vi "view variant in tree helper.vi"(4 "is array element?":bool, 5 "is attribute?":bool, 6 "index string":string, 7 "name":string, 8 "error in (no error)":errorcluster, 9 "Item Indent":i32, 10 "Variant":variant, 11 "Items":T1(array[cluster])) -> (0 "error out":errorcluster, 3 "Items out":T1(array[cluster]))   [LabVIEW 2016]
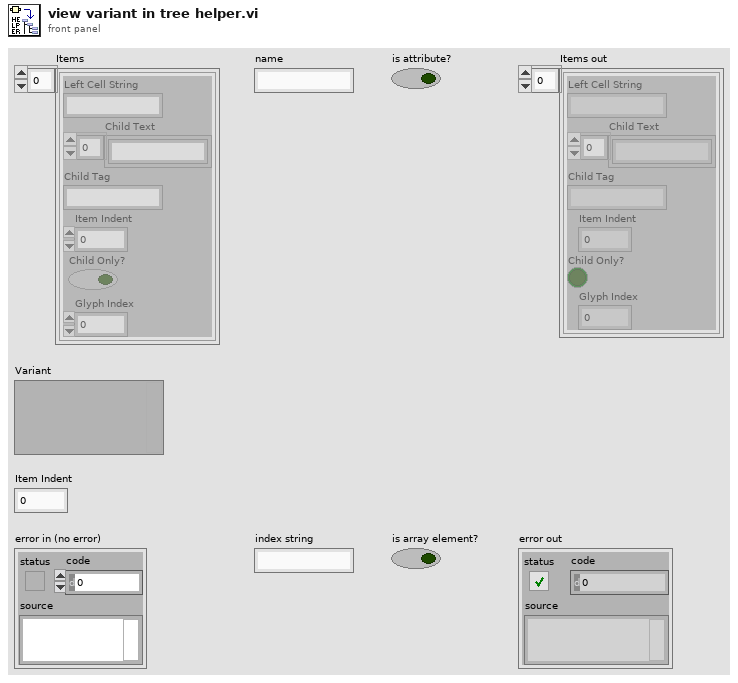
[diagram p1: front panel]
types:
  T1 = cluster{"Left Cell String":string, "Child Text":string[], "Child Tag":string, "Item Indent":i32, "Child Only?":bool, "Glyph Index":i32}[]
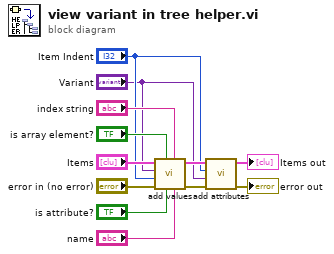
[diagram p0: block diagram]
diagram:
  n1 = call "add values.vi"("name"="name", "index string"="index string", "is attribute?"="is attribute?", "is array element?"="is array element?", "error in (no error)"="error in (no error)", "Item Indent"="Item Indent", "Variant"="Variant", "Items in"="Items") -> ("error out"=w8:errorcluster, "Items out"=w12:T1)  [unwired: 2 in]
  n2 = call "add attributes.vi"("error in (no error)"=w8, "Variant"="Variant", "Item Indent"="Item Indent", "Items in"=w12) -> ("error out"=→"error out":errorcluster, "Items out"=→"Items out":T1)  [unwired: 6 in]
